vi "Merge 2 Cubes.vi"(10 "Cube 1":T2={"X Min"=0, "X Max"=10, "Y Min"=0, "Y Max"=10, "Z Min"=0, "Z Max"=10}, 11 "Cube 2":T2={"X Min"=10, "X Max"=11, "Y Min"=10, "Y Max"=11, "Z Min"=10, "Z Max"=11}) -> (0 "Overlap?":bool, 2 "Cube 1 Parts":T1(array[cluster]), 3 "Cube 2 Parts":T1(array[cluster]))   [LabVIEW 2021]
uses:
  <vilib>/Comparison/Less/Less Functor/Less Functor.lvclass
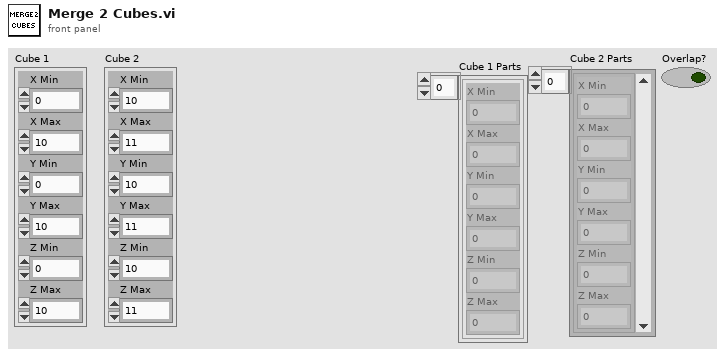
[diagram p1: front panel]
types:
  T1 = cluster{"X Min":i64, "X Max":i64, "Y Min":i64, "Y Max":i64, "Z Min":i64, "Z Max":i64}[]
  T2 = cluster{"X Min":i64, "X Max":i64, "Y Min":i64, "Y Max":i64, "Z Min":i64, "Z Max":i64}
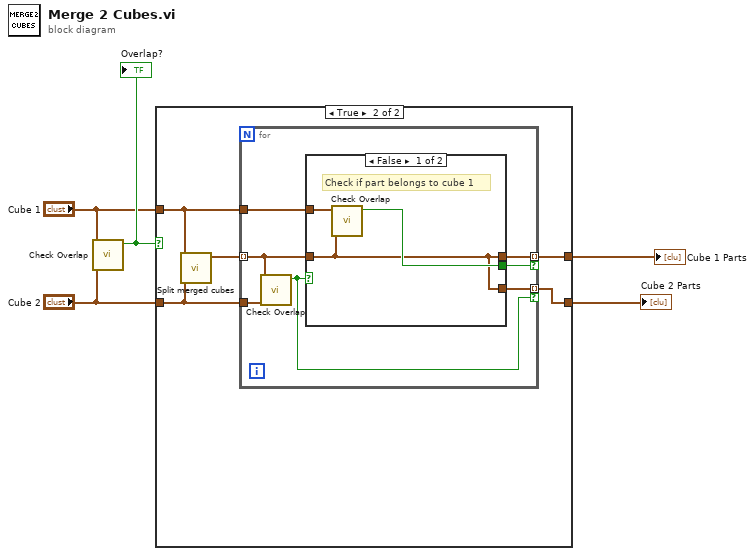
[diagram p0: block diagram]
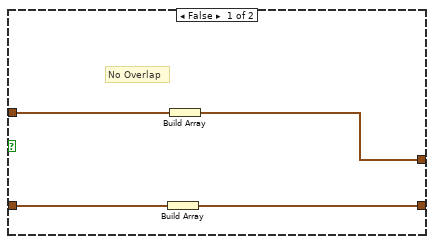
[diagram p2: hidden frame]
diagram:
  n1 = call "Check Overlap.vi"("Cube 2"="Cube 2", "Cube 1"="Cube 1") -> ("Overlap?"=w5:bool)  [unwired: 9 in]
  "Overlap?" <- w5
  n2 = case shown="True" w5 {
    tunnel: "Cube 1" -> [w7 w13]
    tunnel: [w6 w11] -> w2
    tunnel: "Cube 2" -> [w9 w12]
    tunnel: [w8 w10] -> w1
    frame False {
      # "No Overlap"
      n3 = Build Array(w9) -> (w8:T1)
      n4 = Build Array(w7) -> (w6:T1)
    }
    frame True {
      n5 = call "Split merged cubes.vi"("Cube 2"=w12, "Cube 1"=w13) -> ("Splitted Cubes"=w14:T1)  [unwired: 9 in]
      n6 = for {
        tunnel: w14 -> [w20] mode=indexing
        tunnel: w13 -> [w18]
        tunnel: w12 -> [w21]
        tunnel: [w19] -> w11 mode=indexing if=w17
        tunnel: [w16] -> w10 mode=indexing if=w15
        n7 = call "Check Overlap.vi"("Cube 2"=w21, "Cube 1"=w20) -> ("Overlap?"=w15:bool)  [unwired: 9 in]
        n8 = case shown="False" w15 {
          tunnel: w20 -> [w22 w25]
          tunnel: [w22 w25] -> w19
          tunnel: [w23 _] -> w17
          tunnel: w18 -> [w24 _]
          tunnel: [w22 w25] -> w16
          frame False {
            # "Check if part belongs to cube 1"
            n9 = call "Check Overlap.vi"("Cube 2"=w22, "Cube 1"=w24) -> ("Overlap?"=w23:bool)  [unwired: 9 in]
          }
          frame True {
            # "Part belongs to cube 2"
          }
        }
      }
    }
  }
  "Cube 1 Parts" <- w2
  "Cube 2 Parts" <- w1
